vi "DB_Create.vi"() -> ()   [LabVIEW 2020]
uses:
  <vilib>/addons/database/Auxilliary.llb/DB Tools Column Info.ctl
  <vilib>/addons/database/Auxilliary.llb/DB Tools DataTypes.ctl
  <vilib>/addons/database/Connection.llb/DB Tools Open Connec (String).vi
  <vilib>/addons/database/NI_Database_API.lvlib
panel:
  in  "column information":T1[](array[typedef])=[{"column name"="Nom", "data type"=enum."String", "size"=50, "allow null?"=FALSE}, {"column name"="Prénom", "data type"=enum."String", "size"=50, "allow null?"=FALSE}, {"column name"="age", "data type"=enum."Single (SGL)", "size"=0, "allow null?"=FALSE}, {"column name"="Sexe", "data type"=enum."String", "size"=1, "allow null?"=FALSE}, {"column name"="Métier", "data type"=enum."String", "size"=50, "allow null?"=FALSE}, {"column name"="Rémunération", "data type"=enum."Single (SGL)", "size"=0, "allow null?"=FALSE}]
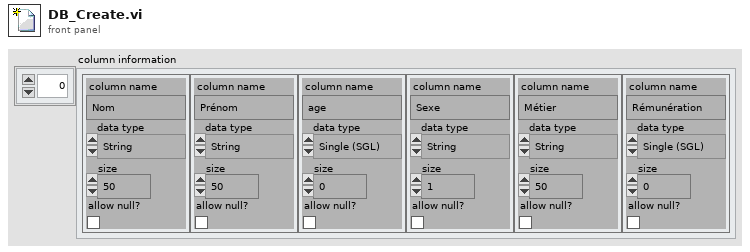
[diagram p1: front panel]
types:
  T1 = typedef "NI_Database_API.lvlib/DB Tools Column Info.ctl" = cluster{"column name":string, "data type":T2, "size":i32, "allow null?":bool}
  T2 = typedef "NI_Database_API.lvlib/DB Tools DataTypes.ctl" = enum16{"String", "Long (I32)", "Single (SGL)", "Double (DBL)", "Date/Time", "Binary"}
  T3 = typedef "NI_Database_API.lvlib/Conn ObjectReference.ctl" = refnum<k1>
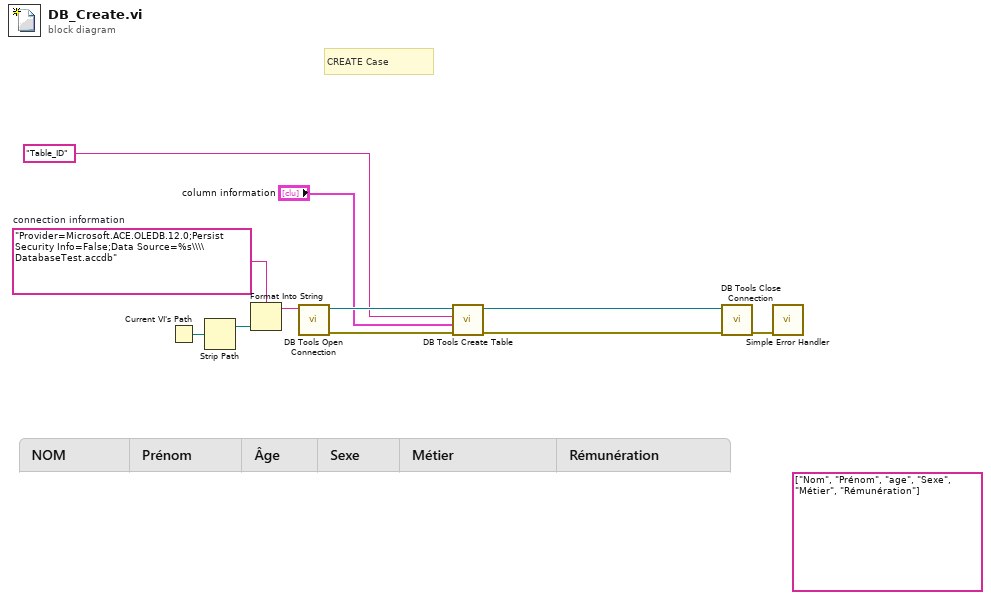
[diagram p0: block diagram]
diagram:
  (unwired) string[] ["Nom", "Prénom", "age", "Sexe", "Métier", "Rémunération"] ("columns")
  w4 = "Provider=Microsoft.ACE.OLEDB.12.0;Persist Security Info=False;Data Source=%s\\\\DatabaseTest.accdb"  # connection information
  # "CREATE Case"
  n1 = Current VI's Path() -> (path=w8:path)
  n2 = Strip Path(path=w8) -> (stripped path=w5:path)  [unwired: 1 out]
  n3 = Format Into String(format string=w4, w5) -> (resulting string=w6:string)  [unwired: 2 in, 1 out]
  n4 = call-poly <vilib>:"DB Tools Open Connection.vi"("connection information"=w6) -> ("error out"=w10:errorcluster, "connection reference"=w11:T3)  [unwired: 7 in]
  n5 = call <vilib>:"DB Tools Create Table.vi"("error in (no error)"=w10, "column information"="column information", "table"="Table_ID", "connection reference"=w11) -> ("error out"=w3:errorcluster, "connection reference out"=w9:T3)  [unwired: 4 in]
  n6 = call <vilib>:"DB Tools Close Connection.vi"("error in (no error)"=w3, "connection reference"=w9) -> ("error out"=w7:errorcluster)  [unwired: 5 in]
  n7 = call <vilib>:"Simple Error Handler.vi"("error in (no error)"=w7) -> ()  [unwired: 4 in, 5 out]
